vi "Get Valve Mode.vi"(8 "error in (no error)":errorcluster, 11 "RRG in":refnum<class "Eltochpribor RRG.lvclass">) -> (0 "error out":errorcluster, 2 "valve mode":u8(ring) items=["auto", "open", "closed"], 3 "RRG out":refnum<class "Eltochpribor RRG.lvclass">)   [LabVIEW 2015, in "Eltochpribor RRG.lvclass"]
doc: "Gets valve mode (automatic flow regulation/open/closed)."
uses:
  Eltochpribor RRG.lvclass
  Modbus Client/PL Modbus Client.lvclass
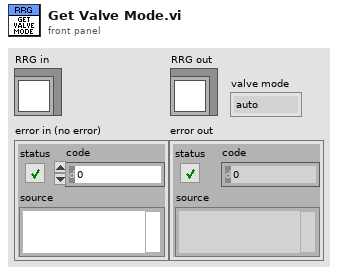
[diagram p1: front panel]
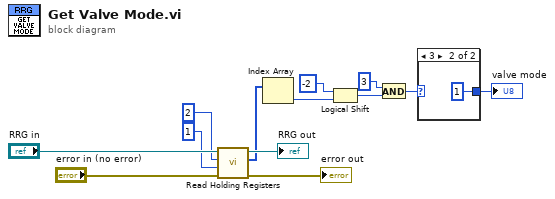
[diagram p0: block diagram]
diagram:
  n1 = call "Read Holding Registers.vi"("error in (no error)"="error in (no error)", "number of holding registers"=u16 1, "address"=u16 2, "MODBUS in"="RRG in") -> ("error out"=→"error out":errorcluster, "values"=w7:u16[], "MODBUS out"=→"RRG out":refnum<class "Eltochpribor RRG.lvclass">)  [unwired: 5 in]
  n2 = Index Array(array=w7) -> (element=w6:u16)  [unwired: 1 in]
  n3 = Logical Shift(y=i16 -2, x=w6) -> (x << y=w4:u16)
  n4 = And(x=u16 3, y=w4) -> (x .and. y?=w2:u16)
  n5 = case shown="3" w2 {
    selector: w2 -> [w14 _]
    tunnel: [w14 u8 1] -> w1
    frame 0, Default {
    }
    frame 3 {
    }
  }
  "valve mode" <- w1
